vi "Build Message Instructions.vi"(7 "Virtual Memory Unit in":refnum<class "Virtual Memory Unit.lvclass">, 8 "error in (no error)":errorcluster, 10 "Starting Address":u16 format="%04x", 11 "Message in":refnum<class "Message.lvclass">) -> (0 "error out":errorcluster, 2 "Next Available Address":u16 format="%04x", 3 "Message out":refnum<class "Message.lvclass">, 5 "Virtual Memory Unit out":refnum<class "Virtual Memory Unit.lvclass">)   [LabVIEW 2020, in "BCI-1553 API.lvlib" / "Message.lvclass"]
doc: "<DO NOT CALL>\n\nA Message doesn't really have 'instructions' of its own. This is really just a call that builds the configuration and data fields into the appropriate memory locations.\n\nAdditionally, it will update it's local parameter list and provide valid linkage addresses for the corresponding parameters. These parameters will be retrieved by the bus controller at a later point for LUT updating."
uses:
  Message.lvclass
  Dependencies/Virtual Memory Unit/Virtual Memory Unit.lvclass
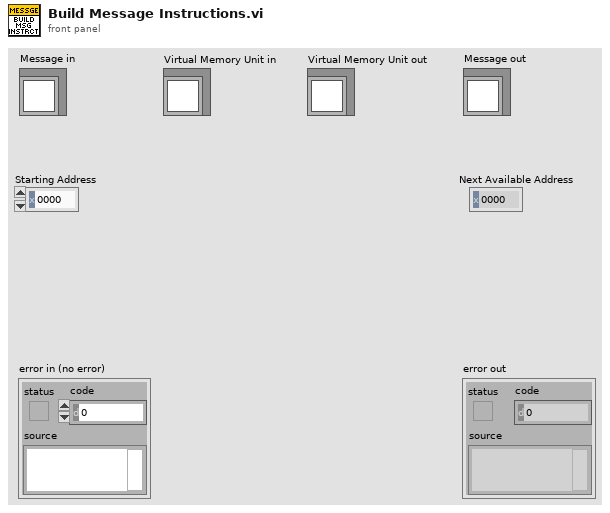
[diagram p1: front panel]
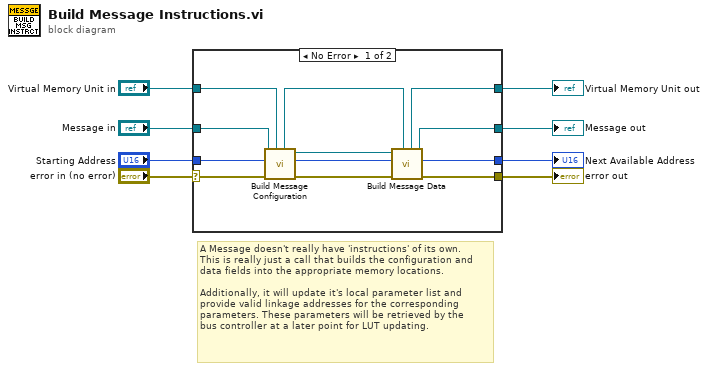
[diagram p0: block diagram]
diagram:
  # "A Message doesn't really have 'instructions' of its own.\nThis is really just a call that builds the configuration and\ndata fields into the appropriate memory locations.\n\nAdditionally, it will update it's local parameter list and\nprovide valid linkage addresses for the corresponding\nparameters. These parameters will be retrieved by the\nbus controller at a later point for LUT updating."
  n1 = case shown="No Error" "error in (no error)" {
    selector: "error in (no error)" -> [w18 w24]
    tunnel: [w9 w24] -> w7
    tunnel: [w11 w23] -> w5
    tunnel: "Message in" -> [w19 w23]
    tunnel: "Virtual Memory Unit in" -> [w17 w21]
    tunnel: "Starting Address" -> [w20 w22]
    tunnel: [w15 w21] -> w2
    tunnel: [w13 w22] -> w1
    frame No Error {
      n2 = call-dynamic "Build Message Configuration.vi"("Virtual Memory Unit in"=w17, "error in (no error)"=w18, "Starting Address"=w20, "Message in"=w19) -> ("error out"=w10:errorcluster, "Next Available Address"=w14:u16, "Message out"=w12:refnum<class "Message.lvclass">, "Virtual Memory Unit out"=w16:refnum<class "Virtual Memory Unit.lvclass">)  [unwired: 4 in]
      n3 = call-dynamic "Build Message Data.vi"("Virtual Memory Unit in"=w16, "error in (no error)"=w10, "Starting Address"=w14, "Message in"=w12) -> ("error out"=w9:errorcluster, "Next Available Address"=w13:u16, "Message out"=w11:refnum<class "Message.lvclass">, "Virtual Memory Unit out"=w15:refnum<class "Virtual Memory Unit.lvclass">)  [unwired: 4 in]
    }
    frame Error {
    }
  }
  "error out" <- w7
  "Message out" <- w5
  "Virtual Memory Unit out" <- w2
  "Next Available Address" <- w1
